vi "IMAQController.AddCameraToCameraList.vi"(0 "i ref in":refnum<vi>, 2 "CS Camera Name":string, 5 "error in (no error)":errorcluster) -> (14 "i ref out":refnum<vi>, 16 "actItem Number":i32[](array[numeric]), 17 "Item Names":string[][](array[string]), 19 "error out":errorcluster)   [LabVIEW 2014, in "IMAQController.lvlib"]
uses:
  IMAQController.lvlib
  CSCore/CSSystem/CoreLib/CoreLib.int 2 byte array.vi
  CSCore/CSSystem/CoreLib/CoreLib.byte array 2 int.vi
  CSCore/CSSystem/CoreLib/CoreLib.byte array 2 double.vi
  CSCore/CSSystem/CoreLib/CoreLib.byte array 2 string.vi
  CSlibraries-extern/DimLVEvent/LVDimInterface/LVDimInterface.lvlib
  CSCore/BaseProcess/BaseProcess.lvlib
  CSCore/CSSystem/CoreLib/CoreLib.lvlib
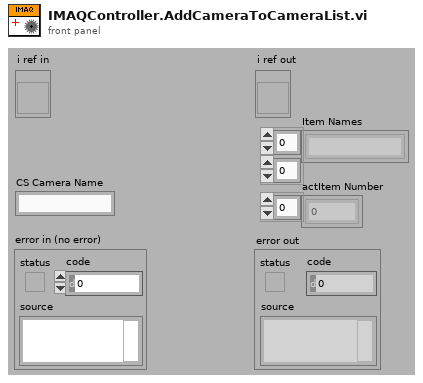
[diagram p1: front panel]
types:
  T1 = cluster{"Grid":cluster{"1":cluster{i32, i32}, "2":cluster{i32, i32}, "3":cluster{i32, i32}, "4":cluster{i32, i32}}, "GridR":cluster{"1":cluster{dbl, dbl}, "2":cluster{dbl, dbl}, "3":cluster{dbl, dbl}, "4":cluster{dbl, dbl}}}
  T2 = typedef "CoreDefs.rawDataType.ctl" = i8[]
  T3 = typedef "CoreDefs.call_type.ctl" = cluster{"Object":string, "Selector":string, "CallType":enum16{"simple", "synchronous", "asynchronous"}, "Async Object":string, "Async Selector":string, "Data Descriptor":T4, "Data":T2, "Error #":i32, "Expire":u32}
  T4 = typedef "BaseProcess.lvlib/BaseProcess.descriptor string definition.ctl" = string
  T5 = cluster{"1":cluster{i32, i32}, "2":cluster{i32, i32}, "3":cluster{i32, i32}, "4":cluster{i32, i32}}
  T6 = cluster{"1":cluster{dbl, dbl}, "2":cluster{dbl, dbl}, "3":cluster{dbl, dbl}, "4":cluster{dbl, dbl}}
  T7 = typedef "IMAQController.lvlib/IMAQController.i attribute.ctl" = cluster{"ImageTakenID":i32, "actSequencer":string, "actScanner":string, "CameraTriggerID":i32, "activatedCameras":cluster{"Name":string, "Camera Type":string, "Acquisition Mode":u32, "JPEG Mode?":bool, "Acquisition Delay":dbl, "Save Images?":bool, "Center Coordinates":T8, "PixelPermm":cluster{"Horizontal":dbl, "Vertical":dbl}, "Rotation":dbl, "Mirror Mode":u32, "PixelCoordinates":cluster{"1":cluster{"Horizontal":i32, "Vertical":i32}, "2":cluster{"Horizontal":i32, "Vertical":i32}, "3":cluster{"Horizontal":i32, "Vertical":i32}, "4":cluster{"Horizontal":i32, "Vertical":i32}}, "RWCoordinates":cluster{"1":cluster{"Horizontal":dbl, "Vertical":dbl}, "2":cluster{"Horizontal":dbl, "Vertical":dbl}, "3":cluster{"Horizontal":dbl, "Vertical":dbl}, "4":cluster{"Horizontal":dbl, "Vertical":dbl}}, "HorizScaling":dbl, "VertScaling":dbl}[], "Ini C-Array":string[], "actCamera":string, "activeCamera":cluster{"Name":string, "Camera Type":string, "Aqcuisation Mode":enum32{"Internal Trigger", "Scan", "free Running", "External Trigger"}, "JPEG Mode?":bool, "Acquisition Delay":dbl, "Save Images?":bool, "Center Coordinates":T8, "PixelPermm":cluster{"Horizontal":dbl, "Vertical":dbl}, "Rotation":dbl, "Mirror Mode":u32, "PixelCoordinates":cluster{"1":cluster{"Horizontal":i32, "Vertical":i32}, "2":cluster{"Horizontal":i32, "Vertical":i32}, "3":cluster{"Horizontal":i32, "Vertical":i32}, "4":cluster{"Horizontal":i32, "Vertical":i32}}, "RWCoordinates":cluster{"1":cluster{"Horizontal":dbl, "Vertical":dbl}, "2":cluster{"Horizontal":dbl, "Vertical":dbl}, "3":cluster{"Horizontal":dbl, "Vertical":dbl}, "4":cluster{"Horizontal":dbl, "Vertical":dbl}}, "HorizScaling":dbl, "VertScaling":dbl}, "BilderMittelungen":u8, "OldPicture":dbl[][]}
  T8 = typedef "LVPoint32TypeDef.ctl" = cluster{"Horizontal":i32, "Vertical":i32}
  T9 = cluster{"CS Camera Name":string, string, u32, bool, dbl, bool, cluster{"i32":i32, "i32":i32}, cluster{"d64":dbl, "d64":dbl}, "d64":dbl, "i32":i32, "Grid":cluster{"1":cluster{i32, i32}, "2":cluster{i32, i32}, "3":cluster{i32, i32}, "4":cluster{i32, i32}}, "GridR":cluster{"1":cluster{dbl, dbl}, "2":cluster{dbl, dbl}, "3":cluster{dbl, dbl}, "4":cluster{dbl, dbl}}, dbl, dbl}
  T10 = cluster{"Name":string, "Camera Type":string, "Acquisition Mode":u32, "JPEG Mode?":bool, "Acquisition Delay":dbl, "Save Images?":bool, "Center Coordinates":T8, "PixelPermm":cluster{"Horizontal":dbl, "Vertical":dbl}, "Rotation":dbl, "Mirror Mode":u32, "PixelCoordinates":cluster{"1":cluster{"Horizontal":i32, "Vertical":i32}, "2":cluster{"Horizontal":i32, "Vertical":i32}, "3":cluster{"Horizontal":i32, "Vertical":i32}, "4":cluster{"Horizontal":i32, "Vertical":i32}}, "RWCoordinates":cluster{"1":cluster{"Horizontal":dbl, "Vertical":dbl}, "2":cluster{"Horizontal":dbl, "Vertical":dbl}, "3":cluster{"Horizontal":dbl, "Vertical":dbl}, "4":cluster{"Horizontal":dbl, "Vertical":dbl}}, "HorizScaling":dbl, "VertScaling":dbl}[]
  T11 = cluster{"CS Camera Name":string, "Camera Type":string, "Acquisition Mode":u32, "JPEG Mode?":bool, "Acquisition Delay":dbl, "Save Images?":bool, "Center Coordinates":T8, "PixelPermm":cluster{"d64":dbl, "d64":dbl}, "d64":dbl, "Mirror Mode":u32, "Grid":cluster{"1":cluster{"Horizontal":i32, "Vertical":i32}, "2":cluster{"Horizontal":i32, "Vertical":i32}, "3":cluster{"Horizontal":i32, "Vertical":i32}, "4":cluster{"Horizontal":i32, "Vertical":i32}}, "GridR":cluster{"1":cluster{"Horizontal":dbl, "Vertical":dbl}, "2":cluster{"Horizontal":dbl, "Vertical":dbl}, "3":cluster{"Horizontal":dbl, "Vertical":dbl}, "4":cluster{"Horizontal":dbl, "Vertical":dbl}}, "HorizScaling":dbl, "VertScaling":dbl}[]
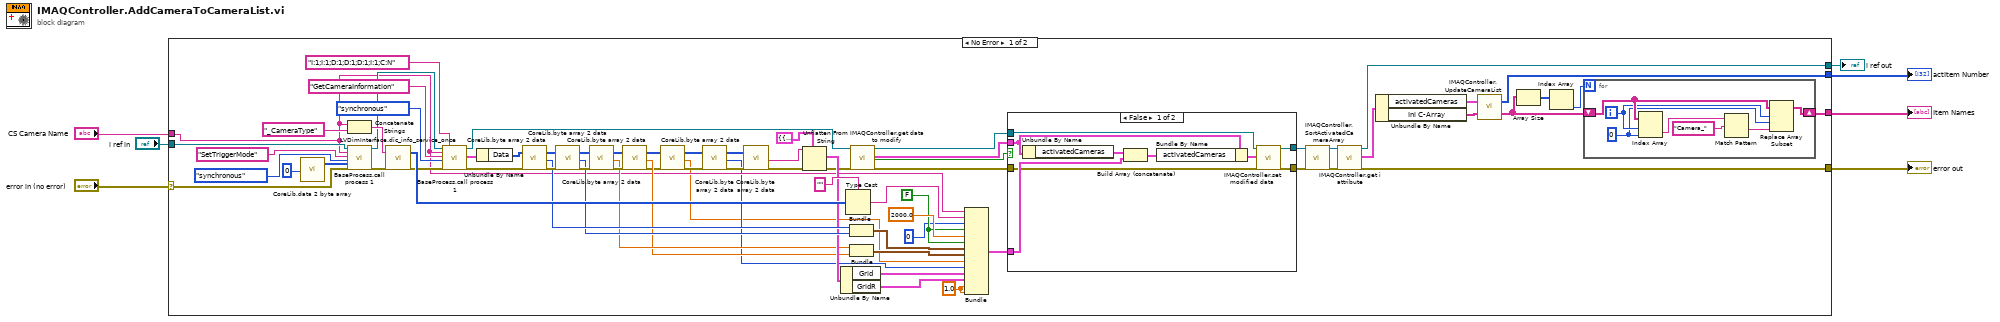
[diagram p0: block diagram]
diagram:
  n1 = case shown="No Error" "error in (no error)" {
    selector: "error in (no error)" -> [w38 w99]
    tunnel: [w25 w98] -> w7
    tunnel: [w24 w99] -> w6
    tunnel: "CS Camera Name" -> [w34 _]
    tunnel: "i ref in" -> [w36 w98]
    tunnel: [w17 _] -> w2
    tunnel: [w16 _] -> w1
    frame No Error {
      w49 = 1.0
      w57 = FALSE
      n2 = call-poly "CoreLib.data 2 byte array.vi"("i32"=0) -> ("byteArray out"=w32:T2)  [unwired: 18 in]
      n3 = Concatenate Strings(w34, "_CameraType" ("string")) -> (w79:string)
      n4 = call "BaseProcess.call process 1.vi"("i ref in"=w36, "Object"=w34, "Selector"="SetTriggerMode", "CallType"=enum16{"simple", "synchronous", "asynchronous"}."synchronous", "Data"=w32, "error in (no error)"=w38) -> ("i ref out"=w35:refnum<vi>, "error out"=w37:errorcluster)  [unwired: 11 in, 1 out]
      n5 = call "LVDimInterface.dic_info_service_once.vi"("serviceName"=w79, "error in (no error)"=w37) -> ("data"=w78:i8[], "error out"=w75:errorcluster)  [unwired: 14 in, 2 out]
      n6 = call "BaseProcess.call process 1.vi"("i ref in"=w35, "Object"=w34, "Selector"="GetCameraInformation", "CallType"=enum16{"simple", "synchronous", "asynchronous"}."synchronous", "error in (no error)"=w75, "Data Descriptor"="I:1;I:1;D:1;D:1;D:1;I:1;C:N") -> ("i ref out"=w40:refnum<vi>, "call cluster out"=w66:T3, "error out"=w64:errorcluster)  [unwired: 11 in]
      n7 = Unbundle By Name(w66) -> ("Data"=w65:T2)
      n8 = call-poly "CoreLib.byte array 2 data.vi"("byteArray"=w65, "error in (no error)"=w64) -> ("byteArray out"=w67:T2, "i32"=w56:i32, "error out"=w63:errorcluster)  [unwired: 15 in]
      n9 = call-poly "CoreLib.byte array 2 data.vi"("byteArray"=w67, "error in (no error)"=w63) -> ("byteArray out"=w68:T2, "i32"=w55:i32, "error out"=w62:errorcluster)  [unwired: 15 in]
      n10 = call-poly "CoreLib.byte array 2 data.vi"("byteArray"=w68, "error in (no error)"=w62) -> ("byteArray out"=w69:T2, "d64"=w48:dbl, "error out"=w61:errorcluster)  [unwired: 15 in]
      n11 = call-poly "CoreLib.byte array 2 data.vi"("byteArray"=w69, "error in (no error)"=w61) -> ("byteArray out"=w12:T2, "d64"=w47:dbl, "error out"=w10:errorcluster)  [unwired: 15 in]
      n12 = call-poly "CoreLib.byte array 2 data.vi"("byteArray"=w12, "error in (no error)"=w10) -> ("byteArray out"=w11:T2, "d64"=w8:dbl, "error out"=w9:errorcluster)  [unwired: 15 in]
      n13 = call-poly "CoreLib.byte array 2 data.vi"("byteArray"=w11, "error in (no error)"=w9) -> ("byteArray out"=w15:T2, "i32"=w13:i32, "error out"=w14:errorcluster)  [unwired: 15 in]
      n14 = call-poly "CoreLib.byte array 2 data.vi"("byteArray"=w15, "error in (no error)"=w14) -> ("string"=w70:string, "error out"=w60:errorcluster)  [unwired: 15 in, 1 out]
      n15 = Unflatten From String(type=T1 {"Grid"={"1"={0, 0}, "2"={0, 0}, "3"={0, 0}, "4"={0, 0}}, "GridR"={"1"={0.0, 0.0}, "2"={0.0, 0.0}, "3"={0.0, 0.0}, "4"={0.0, 0.0}}} ("output cluster"), binary string=w70, error in (no error)=w60) -> (value=w52:T1, error out=w43:errorcluster)  [unwired: 2 in, 1 out]
      n16 = Unbundle By Name(w52) -> ("Grid"=w51:T5, "GridR"=w50:T6)
      n17 = Type Cast(type="", x=w78) -> (*(type *) &x=w59:string)
      n18 = Bundle("i32"=w56, "i32"=w55) -> (w54:cluster{"i32":i32, "i32":i32})  [unwired: 1 in]
      n19 = Bundle("d64"=w48, "d64"=w47) -> (w46:cluster{"d64":dbl, "d64":dbl})  [unwired: 1 in]
      n20 = call "IMAQController.get data to modify.vi"("i ref in"=w40, "error in (no error)"=w43) -> ("i ref out"=w41:refnum<vi>, "i attribute"=w44:T7, "timed out"=w39:bool, "error out"=w42:errorcluster)  [unwired: 14 in]
      n21 = Bundle("CS Camera Name"=w34, w59, u32 0, w57, 2000.0, w57, w54, w46, "d64"=w8, "i32"=w13, "Grid"=w51, "GridR"=w50, w49, w49) -> (w45:T9)  [unwired: 1 in]
      n22 = case shown="False" w39 {
        tunnel: w45 -> [w94 _]
        tunnel: w44 -> [w93 _]
        tunnel: w42 -> [w91 w96]
        tunnel: w41 -> [w90 w97]
        tunnel: [w89 w97] -> w28
        tunnel: [w88 w96] -> w29
        frame False {
          n23 = Unbundle By Name(w93) -> ("activatedCameras"=w95:T10)
          n24 = Build Array (concatenate)(w95, w94) -> (w87:T11)
          n25 = Bundle By Name(cluster=w93, "activatedCameras"=w87) -> (w92:T7)
          n26 = call "IMAQController.set modified data.vi"("i ref in"=w90, "i attribute"=w92, "error in (no error)"=w91) -> ("i ref out"=w89:refnum<vi>, "error out"=w88:errorcluster)  [unwired: 15 in]
        }
        frame True {
        }
      }
      n27 = call "IMAQController.SortActivatedCameraArray.vi"("i ref in"=w28, "error in (no error)"=w29) -> ("i ref out"=w27:refnum<vi>, "error out"=w26:errorcluster)  [unwired: 16 in]
      n28 = call "IMAQController.get i attribute.vi"("i ref in"=w27, "error in (no error)"=w26) -> ("i ref out"=w25:refnum<vi>, "i attribute"=w23:T7, "error out"=w24:errorcluster)  [unwired: 15 in]
      n29 = Unbundle By Name(w23) -> ("activatedCameras"=w19:T10, "Ini C-Array"=w18:string[])
      n30 = call "IMAQController.UpdateCameraList.vi"("activatedCameras"=w19, "Detector.ini List Camera-Array"=w18) -> ("actItem Number"=w16:i32[], "Item Names"=w20:string[][])  [unwired: 16 in]
      n31 = Array Size(array=w20) -> (size(s)=w22:i32[])
      n32 = Index Array(array=w22) -> (element=w21:i32)  [unwired: 1 in]
      n33 = for {
        N: w21 -> [_]
        shift-right: [w80] -> w17
        shift-left: w20 -> [w84]
        i -> [w83]
        w82 = 0 ("disabled index (col)")
        n34 = Index Array(array=w84, index (row)=w83, index (col)=w82) -> (element=w86:string)
        n35 = Match Pattern(string=w86, regular expression="Camera_") -> (after substring=w81:string)  [unwired: 1 in, 3 out]
        n36 = Replace Array Subset(array=w84, new element=w81, index (row)=w83, index (col)=w82) -> (w80:string[][])
      }
    }
    frame Error {
    }
  }
  "i ref out" <- w7
  "error out" <- w6
  "actItem Number" <- w1
  "Item Names" <- w2
